vi "As02.vi"() -> ()   [LabVIEW 2017]
panel:
  in  "stop":bool
  out "LED 5":bool
  in  "x+1 2":i32
  out "x-y*floor(x/y) 2":dbl
  out "floor(x/y) 2":dbl
  in  "y 2":dbl
  out "LED 4":bool
  in  "Knob":dbl(knob) scale=50.0..1000.0
  out "LED 3":bool
  out "LED 2":bool
  in  "x+1":i32
  out "x-y*floor(x/y)":dbl
  out "floor(x/y)":dbl
  in  "y":dbl
  out "LED 1":bool
  out "Boolean":bool
  out "number (0 to 1)":dbl
  out "Thermometer":dbl(slide) scale=0.0..100.0
  out "i ; for":dbl
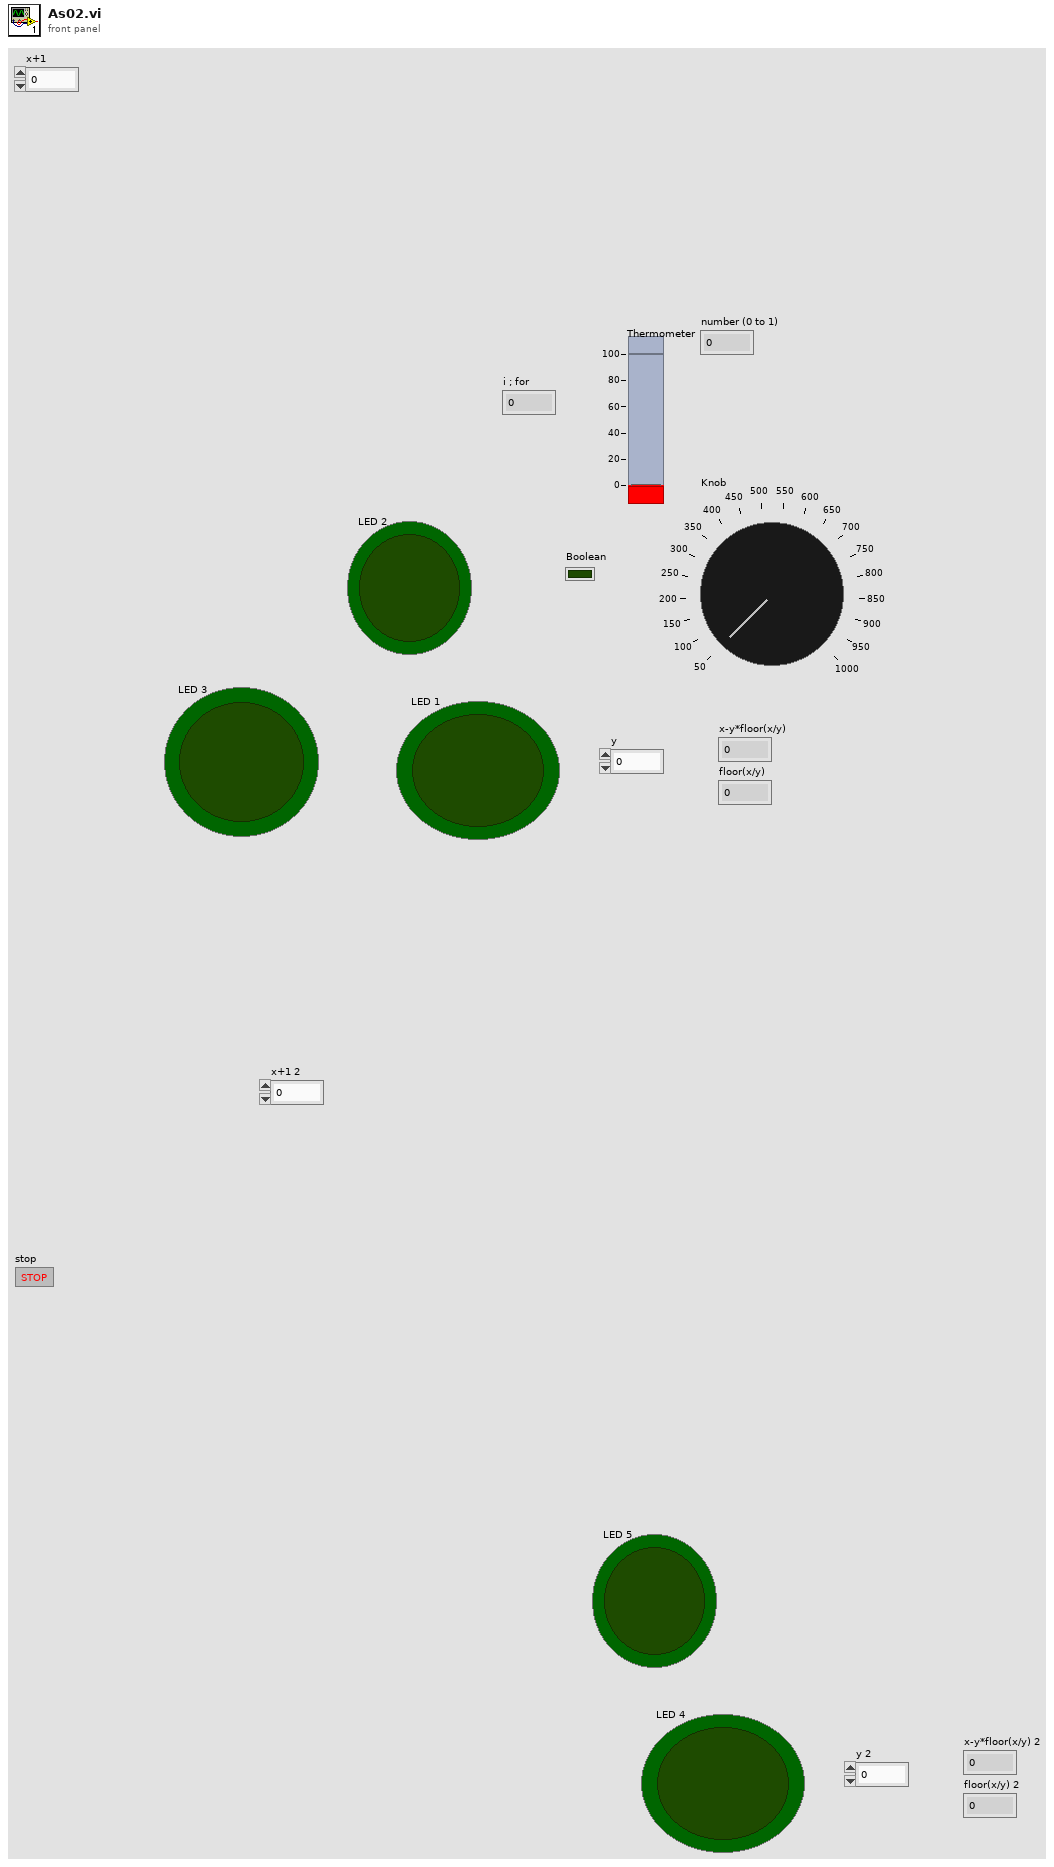
[diagram p1: front panel]
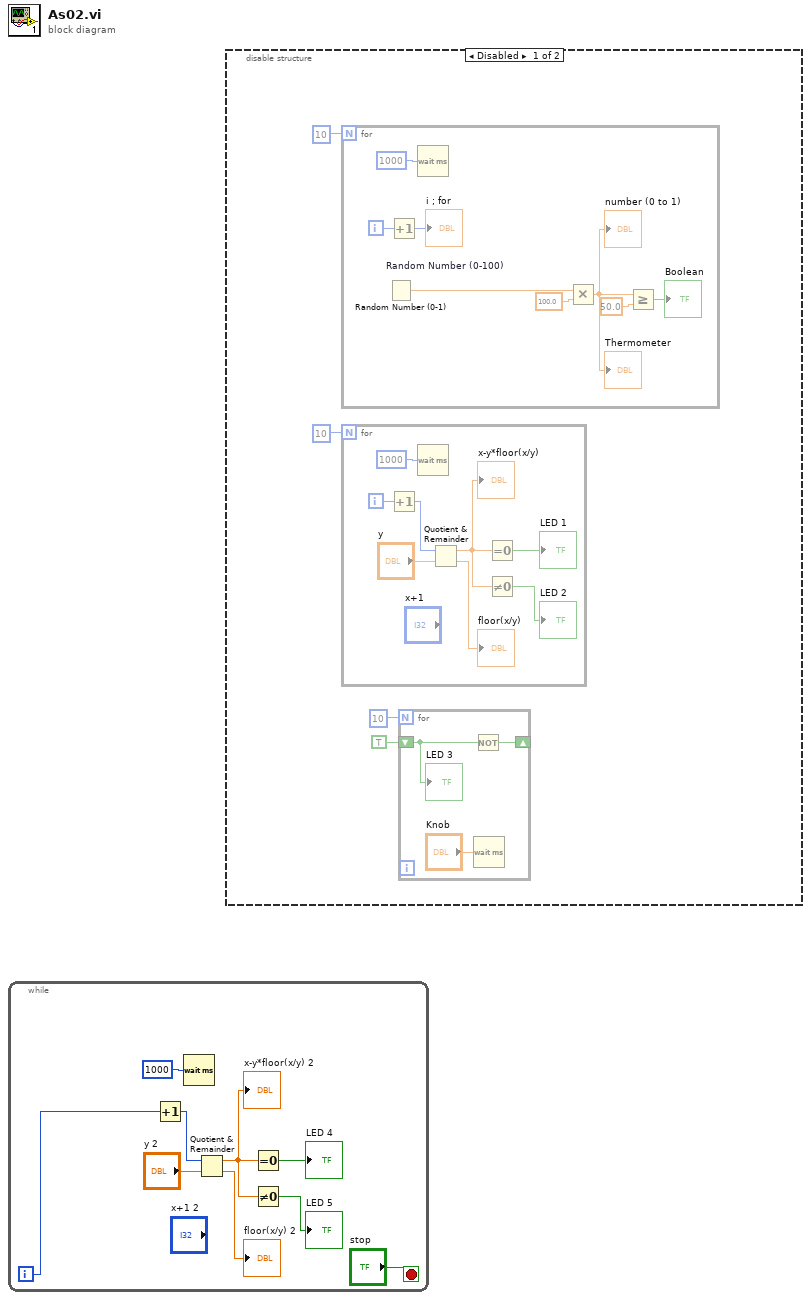
[diagram p0: block diagram]
diagram:
  n1 = while {
    i -> [w1]
    stop <- "stop" stop-if-true
    n2 = Increment(x=w1) -> (x+1=w5:i32)
    n3 = Wait (ms)(milliseconds to wait=u32 1000 ("millisecond timer value")) -> ()  [unwired: 1 out]
    n4 = Quotient & Remainder(x=w5, y="y 2") -> (x-y*floor(x/y)=w2:dbl, floor(x/y)=→"floor(x/y) 2":dbl)
    "x-y*floor(x/y) 2" <- w2
    n5 = Equal To 0?(x=w2) -> (x = 0?=→"LED 4":bool)
    n6 = Not Equal To 0?(x=w2) -> (x != 0?=→"LED 5":bool)
  }
  n7 = disable-structure shown="Disabled" {
    frame Disabled {
      n8 = for {
        N: 10 -> [_]
        i -> [w27]
        n9 = Random Number (0-1) "Random Number (0-100)"() -> (number: 0 to 1=w26:dbl)
        n10 = Increment(x=w27) -> (x+1=→"i ; for":i32)
        n11 = Wait (ms)(milliseconds to wait=u32 1000 ("millisecond timer value")) -> ()  [unwired: 1 out]
        n12 = Multiply(x=w26, y=100.0) -> (x*y=w22:dbl)
        "Thermometer" <- w22
        "number (0 to 1)" <- w22
        n13 = Greater Or Equal?(x=w22, y=50.0) -> (x >= y?=→"Boolean":bool)
      }
      n14 = for {
        N: 10 -> [_]
        i -> [w18]
        n15 = Increment(x=w18) -> (x+1=w17:i32)
        n16 = Wait (ms)(milliseconds to wait=u32 1000 ("millisecond timer value")) -> ()  [unwired: 1 out]
        n17 = Quotient & Remainder(x=w17, y="y") -> (x-y*floor(x/y)=w14:dbl, floor(x/y)=→"floor(x/y)":dbl)
        "x-y*floor(x/y)" <- w14
        n18 = Equal To 0?(x=w14) -> (x = 0?=→"LED 1":bool)
        n19 = Not Equal To 0?(x=w14) -> (x != 0?=→"LED 2":bool)
      }
      n20 = for {
        N: 10 -> [_]
        shift-right: [w31] -> _
        shift-left: TRUE -> [w32]
        n21 = Not(x=w32) -> (.not. x?=w31:bool)
        n22 = Wait (ms)(milliseconds to wait="Knob") -> ()  [unwired: 1 out]
        "LED 3" <- w32
      }
    }
    frame Enabled {
    }
  }
